vi "Initialize OAuth for Google.vi"(6 "Refresh Token":string, 9 "Requested Scopes":string[](array[string])=["email", "profile", "openid"], 10 "Client Secret":string, 11 "Client ID":string) -> (0 "error out":errorcluster, 3 "Oauth2.Google":refnum<class "Oauth2.Google.lvclass">)   [LabVIEW 2017, in "Oauth2.Google.lvclass"]
uses:
  Oauth2.Google.lvclass
  D:/GitHub/Oauth2/source/Oauth2/Oauth2.lvclass
  Oauth2/Oauth2.lvclass
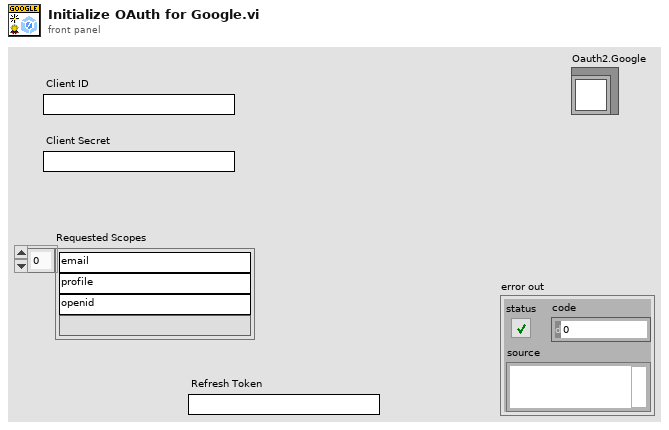
[diagram p1: front panel]
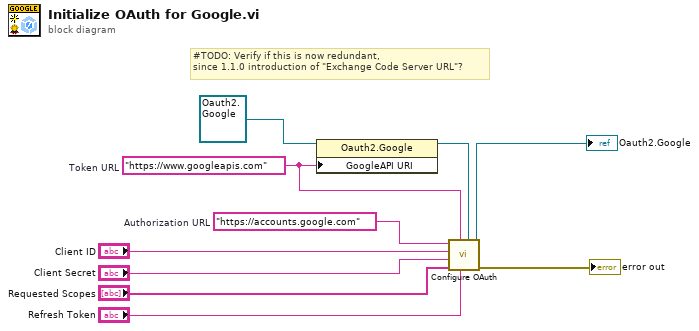
[diagram p0: block diagram]
diagram:
  w5 = "https://accounts.google.com"  # Authorization URL
  w1 = "https://www.googleapis.com"  # Token URL
  # "#TODO: Verify if this is now redundant, \nsince 1.1.0 introduction of \"Exchange Code Server URL\"?"
  n1 = property class="Oauth2.Google"(reference=refnum<class "Oauth2.Google.lvclass"> refnum ("Oauth2.Google.lvclass"), "GoogleAPI URI"=w1) -> (reference out=w2:refnum<class "Oauth2.Google.lvclass">)  [unwired: 1 in, 1 out]
  n2 = call "Configure OAuth.vi"("Oauth2 in"=w2, "Refresh Token"="Refresh Token", "Exchange Code Server URI"=w1, "scopes"="Requested Scopes", "Client Secret"="Client Secret", "Client ID"="Client ID", "Authorization Server URI"=w5) -> ("error out"=→"error out":errorcluster, "Oauth2"=→"Oauth2.Google":refnum<class "Oauth2.Google.lvclass">)  [unwired: 3 in]
